vi "SetROI.vi"(8 "error in (no error)":errorcluster, 10 "Setting.ROI":T1, 11 "Camera_Prime95B in":refnum<class "Camera_Prime95B.lvclass">) -> (0 "error out":errorcluster, 3 "Camera_Prime95B out":refnum<class "Camera_Prime95B.lvclass">)   [LabVIEW 2020, in "Camera_Prime95B.lvlib" / "Camera_Prime95B.lvclass"]
uses:
  Camera_Prime95B.lvclass
  Camera_Prime95B.lvclass/Camera_Prime95B.ctl
  E:/Development/DevHardSoftware/MicroscopyFramework/Model/Hardware Layer/Real Hardware/Camera_Prime95B/Camera_Prime95B/Dependencies/PVCamNET.dll
  Dependencies/PVCamNET.dll
  Controls/Wait For Stop Status.ctl
  Hardware Abstraction Layer/Component/Camera/Camera/Camera.lvclass
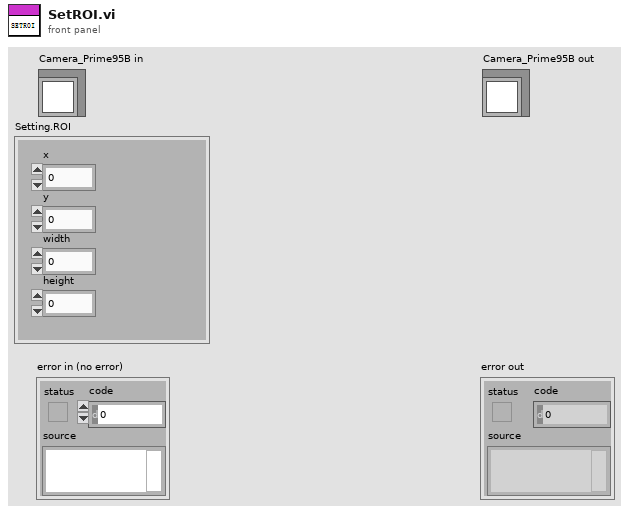
[diagram p1: front panel]
types:
  T1 = cluster{"x":dbl, "y":dbl, "width":dbl, "height":dbl}
  T2 = typedef "Device.lvlib/DeviceStatus.ctl" = i32
  T3 = typedef "Camera.lvlib/Camera.lvclass/Wait For Stop Status.ctl" = i32
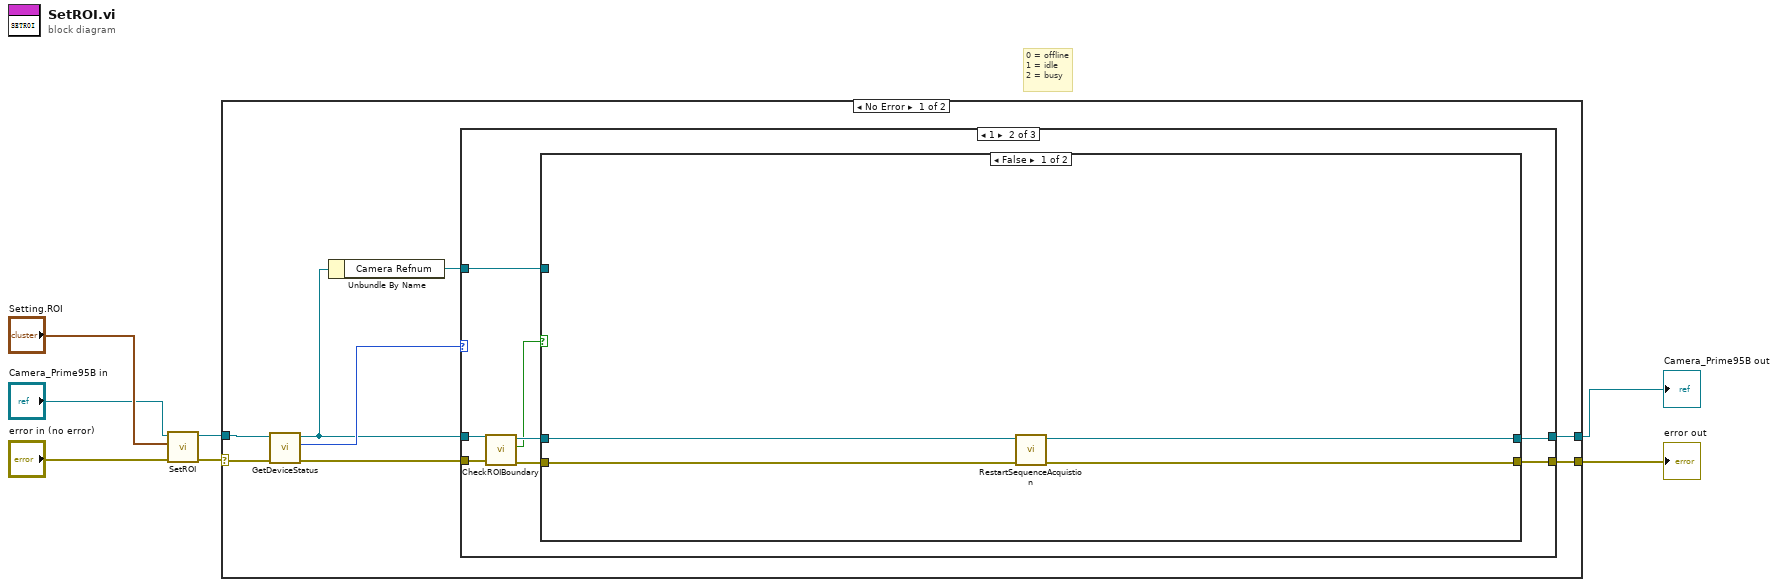
[diagram p0: block diagram]
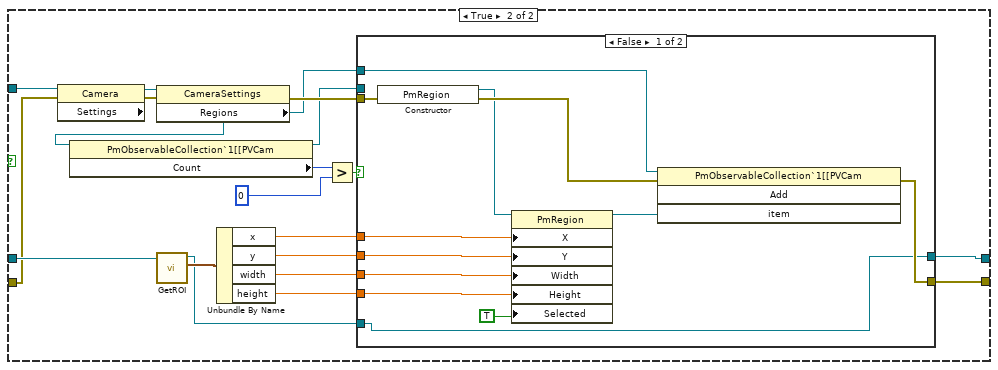
[diagram p3: hidden frame]
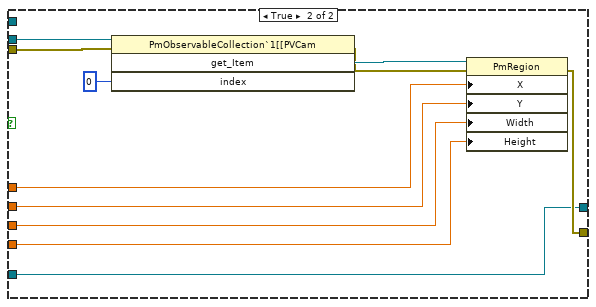
[diagram p4: hidden frame]
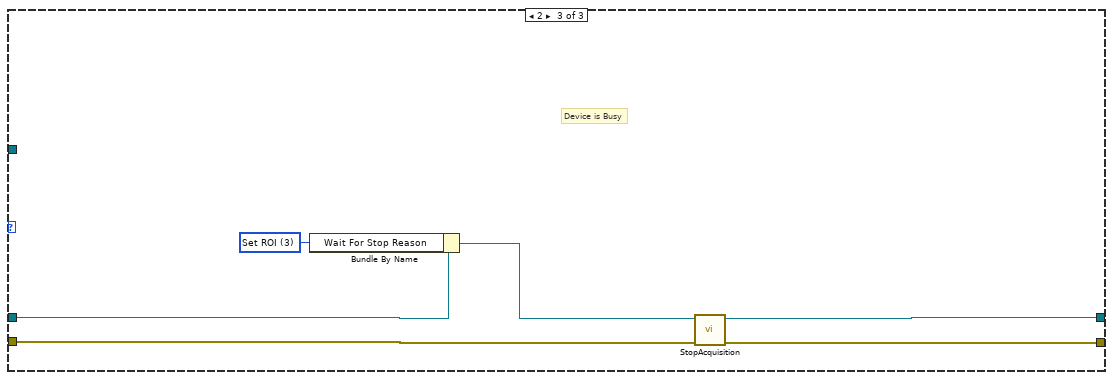
[diagram p5: hidden frame]
diagram:
  # "0 = offline\n1 = idle\n2 = busy"
  n1 = call-parent "SetROI.vi"("error in (no error)"="error in (no error)", "Setting.ROI"="Setting.ROI", "Camera in"="Camera_Prime95B in") -> ("error out"=w4:errorcluster, "Camera out"=w3:refnum<class "Camera_Prime95B.lvclass">)  [unwired: 7 in]
  n2 = case shown="No Error" w4 {
    selector: w4 -> [w14 w79]
    tunnel: [w15 w79] -> w1
    tunnel: w3 -> [w13 w78]
    tunnel: [w10 w78] -> w2
    frame No Error {
      n3 = call-dynamic "GetDeviceStatus.vi"("error in (no error)"=w14, "Camera_Prime95B in"=w13) -> ("error out"=w8:errorcluster, "Status"=w12:T2, "Camera_Prime95B out"=w9:refnum<class "Camera_Prime95B.lvclass">)  [unwired: 7 in]
      n4 = Unbundle By Name(w9) -> ("Camera Refnum"=w11:refnum<k24>)
      n5 = case shown="1" w12 {
        tunnel: [w16 w25 w76] -> w15
        tunnel: w8 -> [w16 w22 w77]
        tunnel: w11 -> [_ w24 _]
        tunnel: w9 -> [w17 w23 w73]
        tunnel: [w17 w18 w74] -> w10
        frame 0, Default {
        }
        frame 1 {
          n6 = call-dynamic "CheckROIBoundary.vi"("error in (no error)"=w22, "Camera in"=w23) -> ("error out"=w20:errorcluster, "Valid?"=w19:bool, "Camera out"=w21:refnum<class "Camera_Prime95B.lvclass">)  [unwired: 7 in]
          n7 = case shown="False" w19 {
            tunnel: [w28 w36] -> w25
            tunnel: w24 -> [_ w34]
            tunnel: w21 -> [w27 w33]
            tunnel: w20 -> [w29 w32]
            tunnel: [w26 w30] -> w18
            frame False {
              n8 = call-dynamic "RestartSequenceAcquistion.vi"("error in (no error)"=w29, "Camera_Prime95B in"=w27) -> ("error out"=w28:errorcluster, "Camera_Prime95B out"=w26:refnum<class "Camera_Prime95B.lvclass">)  [unwired: 8 in]
            }
            frame True {
              n9 = property class="Camera"(reference=w34, error in=w32) -> (error out=w47:errorcluster, "Settings"=w48:refnum<k24>)  [unwired: 1 out]
              n10 = property class="CameraSettings"(reference=w48, error in=w47) -> (error out=w43:errorcluster, "Regions"=w35:refnum<k24>)  [unwired: 1 out]
              n11 = property class="PmObservableCollection`1[[PVCam"(reference=w35) -> (reference out=w42:refnum<k24>, "Count"=w46:i32)  [unwired: 1 in, 1 out]
              n12 = call-dynamic "GetROI.vi"("Camera in"=w33) -> ("Setting.ROI"=w41:T1, "Camera out"=w31:refnum<class "Camera_Prime95B.lvclass">)  [unwired: 8 in, 1 out]
              n13 = Unbundle By Name(w41) -> ("x"=w40:dbl, "y"=w39:dbl, "width"=w38:dbl, "height"=w37:dbl)
              n14 = Greater?(x=w46, y=0) -> (0:w45:bool)
              n15 = case shown="False" w45 {
                tunnel: w42 -> [_ w69]
                tunnel: w43 -> [w57 w68]
                tunnel: [w60 w66] -> w36
                tunnel: w40 -> [w54 w65]
                tunnel: w39 -> [w53 w64]
                tunnel: w38 -> [w52 w63]
                tunnel: w37 -> [w51 w62]
                tunnel: w35 -> [w50 _]
                tunnel: w31 -> [w49 w61]
                tunnel: [w49 w61] -> w30
                frame False {
                  n16 = constructor class="PmRegion"(error in=w57) -> (reference out=w55:refnum<k24>, error out=w56:errorcluster)  [unwired: 2 in, 1 out]
                  n17 = property class="PmRegion"(reference=w55, "X"=w54, "Y"=w53, "Width"=w52, "Height"=w51, "Selected"=TRUE) -> (reference out=w59:refnum<k24>)  [unwired: 1 in, 1 out]
                  n18 = invoke class="PmObservableCollection`1[[PVCam" method="Add"(reference=w50, error in=w56, "item"=w59) -> (error out=w60:errorcluster)  [unwired: 1 in, 3 out]
                }
                frame True {
                  n19 = invoke class="PmObservableCollection`1[[PVCam" method="get_Item"(reference=w69, error in=w68, "index"=0) -> (error out=w67:errorcluster, "get_Item"=w71:refnum<k24>)  [unwired: 1 in, 2 out]
                  n20 = property class="PmRegion"(reference=w71, error in=w67, "X"=w65, "Y"=w64, "Width"=w63, "Height"=w62) -> (error out=w66:errorcluster)  [unwired: 1 out]
                }
              }
            }
          }
        }
        frame 2 {
          w75 = T3 3 items=["None", "Set Exposure", "Set Binning", "Set ROI", "Senquen Acq", ""] ("Wait For Stop Reason")
          # "Device is Busy"
          n21 = Bundle By Name(cluster=w73, "Wait For Stop Reason"=w75) -> (w72:refnum<class "Camera_Prime95B.lvclass">)
          n22 = call-dynamic "StopAcquisition.vi"("error in (no error)"=w77, "Camera_Prime95B in"=w72) -> ("error out"=w76:errorcluster, "Camera_Prime95B out"=w74:refnum<class "Camera_Prime95B.lvclass">)  [unwired: 8 in]
        }
      }
    }
    frame Error {
    }
  }
  "error out" <- w1
  "Camera_Prime95B out" <- w2
